vi "IFile Close.vi"(8 "error in (no error)":errorcluster, 11 "INIScoreFile in":refnum<class "INIScoreFile.lvclass">) -> (0 "error out":errorcluster, 3 "INIScoreFile out":refnum<class "INIScoreFile.lvclass">)   [LabVIEW 2020, in "INIScoreFile.lvclass"]
uses:
  INIScoreFile.lvclass
  INIScoreFile.lvclass/INIScoreFile.ctl
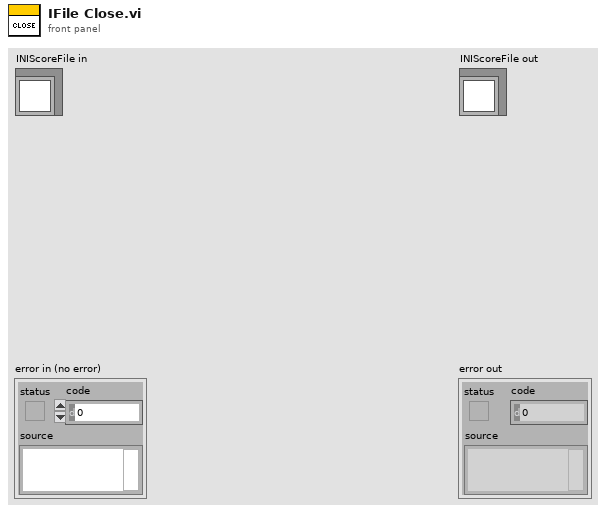
[diagram p1: front panel]
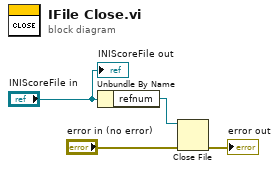
[diagram p0: block diagram]
diagram:
  n1 = Unbundle By Name("INIScoreFile in") -> ("refnum"=w3:refnum<file>)
  n2 = Close File(refnum=w3, error in="error in (no error)") -> (error out=→"error out":errorcluster)  [unwired: 1 out]
  "INIScoreFile out" <- "INIScoreFile in"
